vi "Check and Create Folder.vi"(8 "error in":errorcluster, 10 "Folder Name":string="Flight Logs", 11 "Path to Directory":path) -> (0 "error out":errorcluster, 3 "Path to Folder":path)   [LabVIEW 2014]
panel:
  out "folder names":string[](array[string])
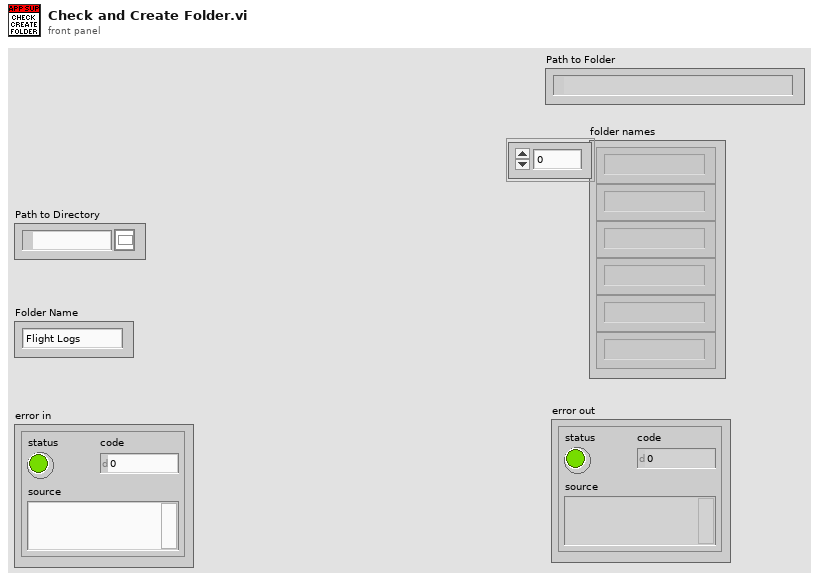
[diagram p1: front panel]
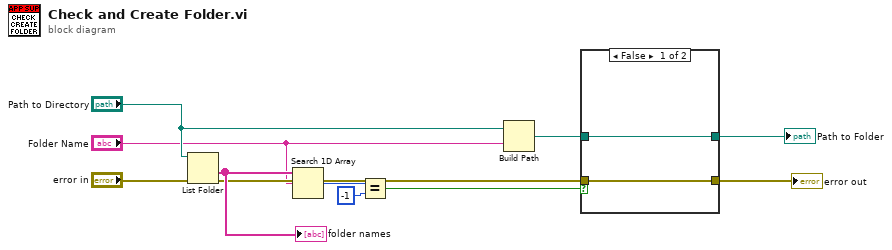
[diagram p0: block diagram]
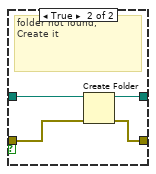
[diagram p2: hidden frame]
diagram:
  n1 = List Folder(path="Path to Directory", error in="error in") -> (folder names=w8:string[], error out=w4:errorcluster)  [unwired: 2 in, 2 out]
  "folder names" <- w8
  n2 = Search 1D Array(1D array=w8, element="Folder Name") -> (index of element=w7:i32)  [unwired: 1 in]
  n3 = Equal?(x=w7, y=-1) -> (x = y?=w5:bool)
  n4 = Build Path(base path="Path to Directory", name or relative path="Folder Name") -> (appended path=w3:path)
  n5 = case shown="False" w5 {
    tunnel: w3 -> [w12 w17]
    tunnel: [w12 w16] -> w11
    tunnel: w4 -> [w13 w15]
    tunnel: [w13 w14] -> w10
    frame False {
    }
    frame True {
      # "folder not found,\nCreate it"
      n6 = Create Folder(path (use dialog)=w17, error in=w15) -> (created path=w16:path, error out=w14:errorcluster)  [unwired: 1 in, 1 out]
    }
  }
  "Path to Folder" <- w11
  "error out" <- w10
